vi "NMLDAQ_periodic_data_backup.vi"() -> ()   [LabVIEW 2020]
uses:
  <vilib>/Utility/file.llb/Write To Spreadsheet File (DBL).vi
panel:
  in  "NML Data Acquisition VI":string(combo)="NML Data Acquisition-New.vi"
  in  "delete backup file\nif original is saved":bool=TRUE
  out "error out":errorcluster
  in  "period (min)":dbl=1.0
  out "time to backup (min)":dbl=0.09166666666666667 format="%#.3g"
  out "last backup":timestamp=timestamp(3589300458.345831 s since 1904-01-01)
  in  "stop":bool
  in  "backup now":bool
  out "Backup file path":path
  out "data":dbl[][](array[numeric])
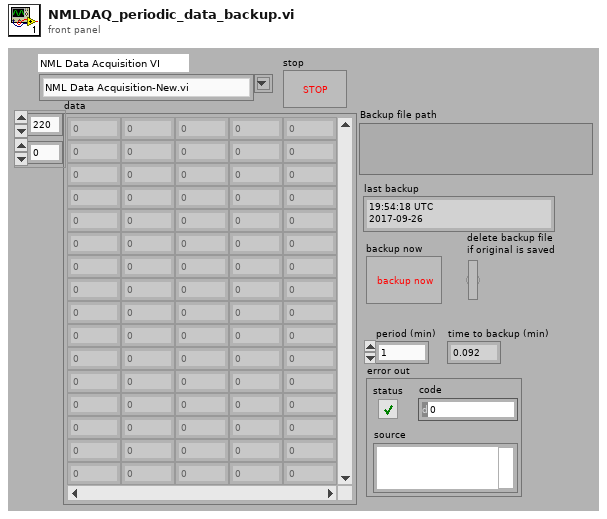
[diagram p1: front panel]
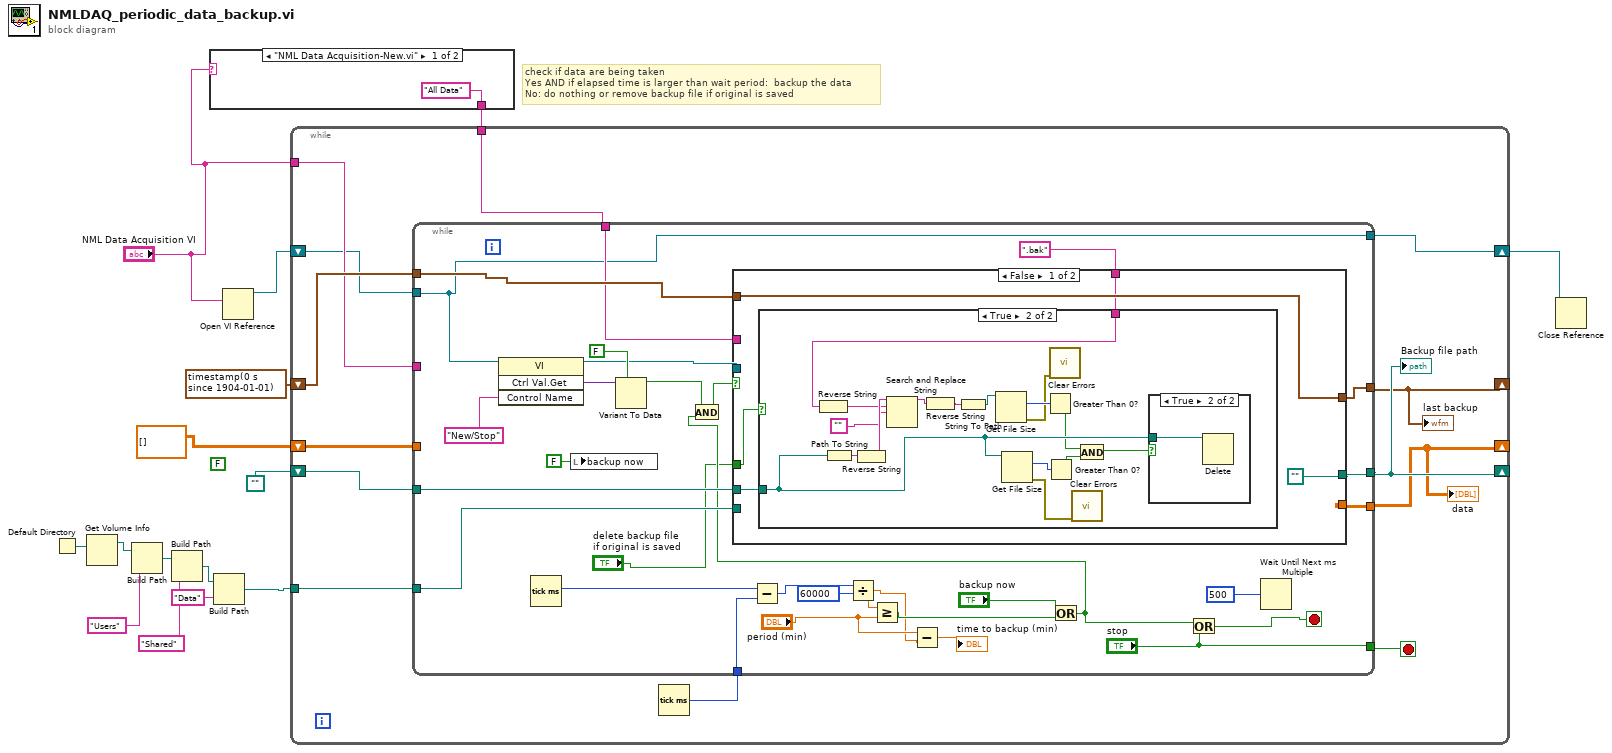
[diagram p0: block diagram]
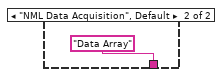
[diagram p2: hidden frame]
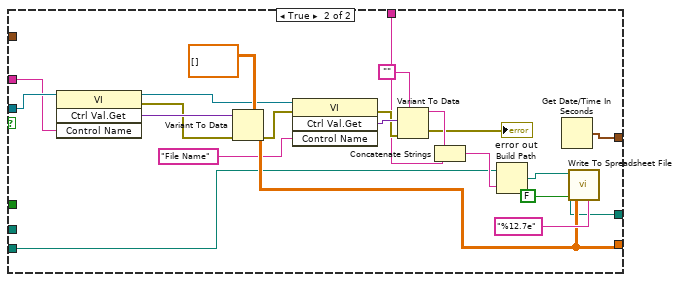
[diagram p5: hidden frame]
diagram:
  (unwired) FALSE ("Periodic backup")
  # "check if data are being taken\nYes AND if elapsed time is larger than wait period:  backup the data\nNo: do nothing or remove backup file if original is saved"
  n1 = Default Directory() -> (w10:path)
  n2 = Get Volume Info(11:w10) -> (5:w9:path)  [unwired: 1 in, 5 out]
  n3 = Build Path(base path=w9, name or relative path="Users") -> (appended path=w11:path)
  n4 = Build Path(base path=w11, name or relative path="Shared") -> (appended path=w8:path)
  n5 = case shown="\"NML Data Acquisition-New.vi\"" "NML Data Acquisition VI" {
    tunnel: ["All Data" ("Control Name") "Data Array" ("Control Name")] -> w4
    frame "NML Data Acquisition-New.vi" {
    }
    frame "NML Data Acquisition", Default {
    }
  }
  n6 = Build Path(base path=w8, name or relative path="Data") -> (appended path=w6:path)
  n7 = Open VI Reference(vi path="NML Data Acquisition VI") -> (vi reference=w3:refnum<vi>)  [unwired: 1 in, 5 out]
  n8 = while {
    shift-right: [w26] -> _
    shift-left: dbl[][] [] ("data") -> [w24]
    shift-right: [w27] -> _
    shift-left: path "" ("new file path (Not A Path if cancelled)") -> [w30]
    shift-right: [w25] -> _
    shift-left: timestamp(0 s since 1904-01-01) ("seconds since 1Jan1904") -> [w23]
    tunnel: w6 -> [w22]
    tunnel: "NML Data Acquisition VI" -> [w21]
    tunnel: w4 -> [w20]
    shift-right: [w18] -> w1
    shift-left: w3 -> [w19]
    stop <- w28 stop-if-true
    n9 = Tick Count (ms)() -> (millisecond timer value=w29:u32)
    n10 = while {
      tunnel: w21 -> [_]
      tunnel: w30 -> [w49]
      tunnel: w29 -> [w59]
      tunnel: ["stop"] -> w28
      tunnel: [w52] -> w26
      tunnel: [w51] -> w25
      tunnel: [w50] -> w27
      tunnel: w24 -> [_]
      tunnel: w23 -> [w48]
      tunnel: w22 -> [w46]
      tunnel: w20 -> [w41]
      tunnel: w19 -> [w31]
      tunnel: [w31] -> w18
      stop <- w54 stop-if-true
      n11 = invoke class="VI" method="Ctrl Val.Get"(reference=w31, "Control Name"="New/Stop") -> (reference out=w37:refnum<vi>, "Get Control Value Variant"=w40:variant)  [unwired: 2 in, 2 out]
      n12 = Tick Count (ms)() -> (millisecond timer value=w60:u32)
      n13 = local write "backup now"(FALSE ("backup now")) -> ()
      n14 = Variant To Data(type=FALSE, Variant=w40) -> (data=w35:bool)  [unwired: 1 in, 1 out]
      n15 = Subtract(x=w60, y=w59) -> (x-y=w58:u32)
      n16 = Divide(x=w58, y=u32 60000) -> (x/y=w44:dbl)
      n17 = Greater Or Equal?(x=w44, y="period (min)") -> (x >= y?=w56:bool)
      n18 = Subtract(x="period (min)", y=w44) -> (x-y=→"time to backup (min)":dbl)
      n19 = Or(x="backup now", y=w56) -> (x .or. y?=w34:bool)
      n20 = And(x=w35, y=w34) -> (x .and. y?=w33:bool)
      n21 = case shown="False" w33 {
        tunnel: [_ w98] -> w52
        tunnel: [w65 w97] -> w51
        tunnel: [path "" w96] -> w50
        tunnel: w46 -> [_ w87]
        tunnel: w48 -> [w65 _]
        tunnel: w37 -> [_ w92]
        tunnel: w49 -> [w62 _]
        tunnel: ".bak" ("string") -> [w63 w85]
        tunnel: w41 -> [_ w84]
        tunnel: "delete backup file\nif original is saved" -> [w61 _]
        frame False {
          n22 = case shown="True" w61 {
            tunnel: w63 -> [_ w78]
            tunnel: w62 -> [_ w72]
            frame False {
            }
            frame True {
              n23 = Reverse String(1:w78) -> (0:w77:string)
              n24 = Path To String(path=w72) -> (string=w81:string)
              n25 = Reverse String(1:w81) -> (0:w80:string)
              n26 = Search and Replace String(input string=w80, search string=w77, replace string="") -> (result string=w76:string)  [unwired: 5 in, 3 out]
              n27 = Reverse String(1:w76) -> (0:w75:string)
              n28 = String To Path(string=w75) -> (path=w74:path)
              n29 = Get File Size(file=w74) -> (size (in bytes)=w73:i64, 0:w67:errorcluster)  [unwired: 1 in, 1 out]
              n30 = Get File Size(file=w72) -> (size (in bytes)=w71:i64, 0:w66:errorcluster)  [unwired: 1 in, 1 out]
              n31 = Greater Than 0?(x=w73) -> (x > 0?=w70:bool)
              n32 = Greater Than 0?(x=w71) -> (x > 0?=w69:bool)
              n33 = call <vilib>:"Clear Errors.vi"("error in (no error)"=w67) -> ()  [unwired: 5 in, 2 out]
              n34 = call <vilib>:"Clear Errors.vi"("error in (no error)"=w66) -> ()  [unwired: 5 in, 2 out]
              n35 = And(x=w70, y=w69) -> (x .and. y?=w68:bool)
              n36 = case shown="True" w68 {
                tunnel: w72 -> [_ w82]
                frame False {
                }
                frame True {
                  n37 = Delete(path (use dialog)=w82) -> ()  [unwired: 4 in, 3 out]
                }
              }
            }
          }
        }
        frame True {
          n38 = invoke class="VI" method="Ctrl Val.Get"(reference=w92, "Control Name"=w84) -> (reference out=w91:refnum<vi>, error out=w90:errorcluster, "Get Control Value Variant"=w94:variant)  [unwired: 2 in, 1 out]
          n39 = Variant To Data(error in=w90, type=dbl[][] [] ("data"), Variant=w94) -> (data=w98:dbl[][], error out=w89:errorcluster)
          n40 = invoke class="VI" method="Ctrl Val.Get"(reference=w91, error in=w89, "Control Name"="File Name") -> (error out=w88:errorcluster, "Get Control Value Variant"=w95:variant)  [unwired: 1 in, 2 out]
          n41 = Variant To Data(error in=w88, type="", Variant=w95) -> (data=w86:string, error out=→"error out":errorcluster)
          n42 = Concatenate Strings(w86, w85) -> (w103:string)
          n43 = Build Path(base path=w87, name or relative path=w103) -> (appended path=w102:path)
          n44 = Get Date/Time In Seconds() -> (seconds since 1Jan1904=w97:timestamp)
          n45 = call-poly <vilib>:"Write To Spreadsheet File.vi"("format (%.3f)"="%12.7e", "append to file? (new file:F)"=FALSE, "2D data"=w98, "file path (dialog if empty)"=w102) -> ("new file path (Not A Path if cancelled)"=w96:path)  [unwired: 2 in, 2 out]
        }
      }
      n46 = Or(x=w34, y="stop") -> (x .or. y?=w54:bool)
      n47 = Wait Until Next ms Multiple(millisecond multiple=u32 500) -> ()  [unwired: 1 out]
    }
    "Backup file path" <- w27
    "data" <- w26
    "last backup" <- w25
  }
  n48 = Close Reference(reference=w1) -> ()  [unwired: 1 in, 1 out]
